vi "Get Test Log Factory.vi"(11 "Model in":refnum<class "Model.lvclass">) -> (2 "Test Log Factory.lvclass":refnum<class "Test Log Factory.lvclass">, 3 "Model out":refnum<class "Model.lvclass">)   [LabVIEW 2015]
uses:
  Model.lvclass
  Test Log/Test Log Factory/Test Log Factory.lvclass
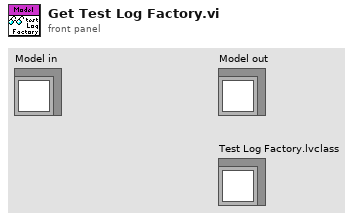
[diagram p1: front panel]
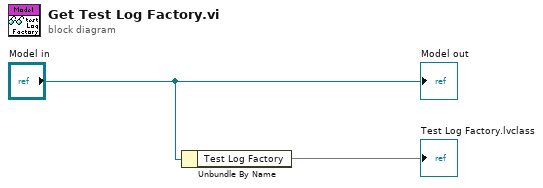
[diagram p0: block diagram]
diagram:
  n1 = Unbundle By Name("Model in") -> ("Test Log Factory"=→"Test Log Factory.lvclass")
  "Model out" <- "Model in"
